vi "Scale RGB Channels of Image Data.vi"(8 "错误输入":errorcluster, 10 "Scale":cluster{"Red":dbl, "Green":dbl, "Blue":dbl} {"Blue" scale=0.0..100.0; "Green" scale=0.0..100.0; "Red" scale=0.0..100.0}, 11 "image data In":T1 caption="输入图像数据") -> (0 "错误输出":errorcluster, 3 "image data Out":T1 caption="输出图像数据")   [LabVIEW 2011]
uses:
  <vilib>/picture/picture.llb/imagedata.ctl
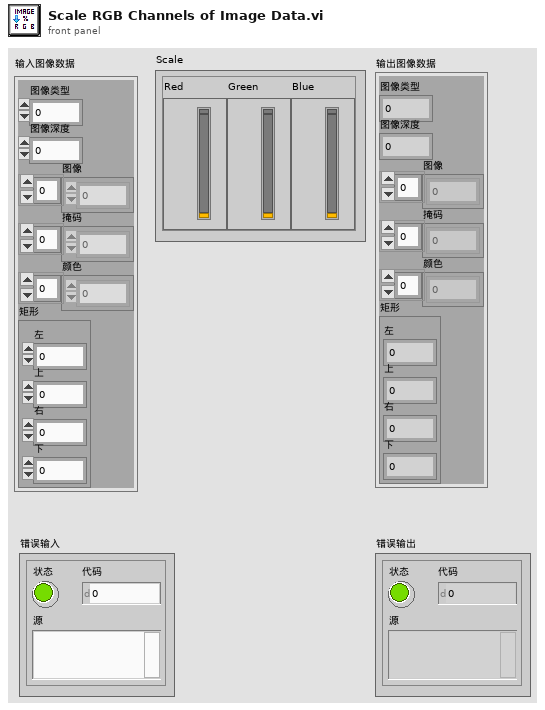
[diagram p1: front panel]
types:
  T1 = typedef "imagedata.ctl" = cluster{"image type":i32, "image depth":i32, "image":u8[], "mask":u8[], "colors":u32[], "Rectangle":cluster{"left":i16, "top":i16, "right":i16, "bottom":i16}}
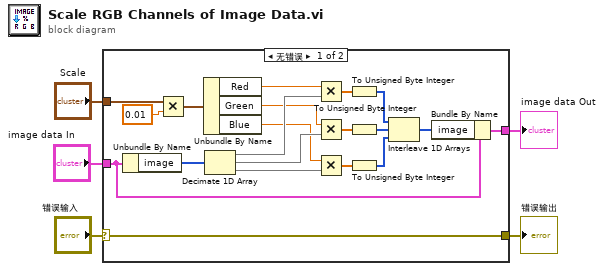
[diagram p0: block diagram]
diagram:
  n1 = case shown="无错误" "错误输入" {
    selector: "错误输入" -> [w23 w26]
    tunnel: "image data In" -> [w25 _]
    tunnel: [w24 _] -> w4
    tunnel: [w23 w26] -> w2
    tunnel: "Scale" -> [w21 _]
    frame No Error {
      n2 = Unbundle By Name(w25) -> ("image"=w22:u8[])
      n3 = Multiply(x=w21, y=0.01) -> (x*y=w19:cluster{"Red":dbl, "Green":dbl, "Blue":dbl})
      n4 = Unbundle By Name(w19) -> ("Red"=w18:dbl, "Green"=w16:dbl, "Blue"=w14:dbl)
      n5 = Decimate 1D Array(w22) -> (w17:u8[], w15:u8[], w13:u8[])
      n6 = Multiply(x=w18, y=w17) -> (x*y=w12:dbl[])
      n7 = Multiply(x=w16, y=w15) -> (x*y=w11:dbl[])
      n8 = Multiply(x=w14, y=w13) -> (x*y=w10:dbl[])
      n9 = To Unsigned Byte Integer(number=w12) -> (unsigned 8bit integer=w9:u8[])
      n10 = To Unsigned Byte Integer(number=w11) -> (unsigned 8bit integer=w8:u8[])
      n11 = To Unsigned Byte Integer(number=w10) -> (unsigned 8bit integer=w7:u8[])
      n12 = Interleave 1D Arrays(w9, w8, w7) -> (w6:u8[])
      n13 = Bundle By Name(cluster=w25, "image"=w6) -> (w24:T1)
    }
    frame Error {
    }
  }
  "image data Out" <- w4
  "错误输出" <- w2
